vi "temp_set_logic.vi"(10 "Write Temperature":dbl=25.0) -> (2 "Read Temperature":dbl)   [LabVIEW 2011]
doc: "This VI sets the the thermal head at any temperature between -15 and 110 degree celsius through the controller.\n\nInputs:\n1. Write Temperature : The required temperature for the thermal head.\n\nOutputs:\n1. Read Temperature : The actual temperature read by the controller.\n2.Error Message: Invalid Temperature (pops up when the user tries to set any temperature which is not in the range)"
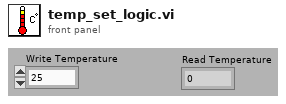
[diagram p1: front panel]
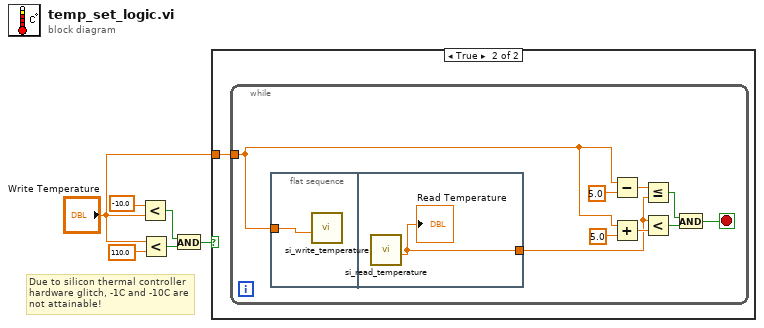
[diagram p0: block diagram]
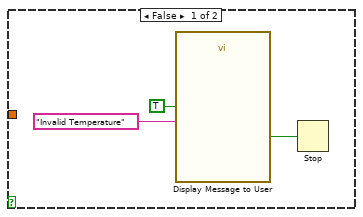
[diagram p2: hidden frame]
diagram:
  # "Due to silicon thermal controller\nhardware glitch, -1C and -10C are\nnot attainable!"
  n1 = Less?(x=-10.0, y="Write Temperature") -> (x < y?=w4:bool)
  n2 = Less?(x="Write Temperature", y=110.0) -> (x < y?=w3:bool)
  n3 = And(x=w4, y=w3) -> (x .and. y?=w2:bool)
  n4 = case shown="True" w2 {
    tunnel: "Write Temperature" -> [_ w10]
    frame False {
      n5 = call "Display Message to User"("Enable"=TRUE, "Message"="Invalid Temperature") -> ("OK"=w7:bool)  [unwired: 8 in, 1 out]
      n6 = Stop(stop? (T)=w7) -> ()
    }
    frame True {
      n7 = while {
        tunnel: w10 -> [w11]
        stop <- w13 stop-if-true
        n8 = flat-sequence {
          tunnel: w11 -> [w20]
          tunnel: [w21] -> w12
          frame #0 {
            n9 = call "si_write_temperature.vi"("INPUT TEMPERATURE"=w20) -> ()  [unwired: 11 in]
          }
          frame #1 {
            n10 = call "si_read_temperature.vi"() -> ("Read Temperature"=w21:dbl)  [unwired: 11 in]
            "Read Temperature" <- w21
          }
        }
        n11 = Subtract(x=w11, y=5.0) -> (x-y=w16:dbl)
        n12 = Add(x=w11, y=5.0) -> (x+y=w15:dbl)
        n13 = Less Or Equal?(x=w16, y=w12) -> (x <= y?=w18:bool)
        n14 = Less?(x=w12, y=w15) -> (x < y?=w14:bool)
        n15 = And(x=w18, y=w14) -> (x .and. y?=w13:bool)
      }
    }
  }
